vi "大项目框外观 1.vi"(0 "Data In":T4 caption="数据输入", 2 "Display State In":T2 caption="显示状态输入", 3 "Container State":T3 caption="容器状态") -> (6 "Data Out":T4 caption="数据输出", 7 "Display State Out":T2 caption="显示状态输出", 8 "Action":T1 caption="动作")   [LabVIEW 2016, in "大项目框.xctl"]
uses:
  <vilib>/_xctls/Container State.ctl
  <vilib>/_xctls/Action.ctl
  <vilib>/_xctls/XControlSupport.lvlib
panel:
  out "单位":string="mg/L"
  out "浓度":string
  out "英文项目名称":string
  out "中文项目名称":string
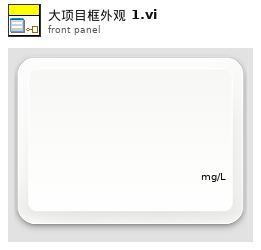
[diagram p1: front panel]
types:
  T1 = typedef "XControlSupport.lvlib/Action.ctl" = cluster{"Data Changed?":bool, "State Changed?":bool, "Action Name":string}
  T2 = typedef "大项目框.xctl/大项目框状态 1.ctl" = cluster{"Numeric":dbl}
  T3 = typedef "XControlSupport.lvlib/Container State.ctl" = cluster{"Indicator?":bool, "Run Mode?":bool, " Refnum":refnum<vi>}
  T4 = typedef "大项目框.xctl/大项目框数据 1.ctl" = cluster{"中文项目名称":string, "英文项目名称":string, "浓度值":string, "单位":string}
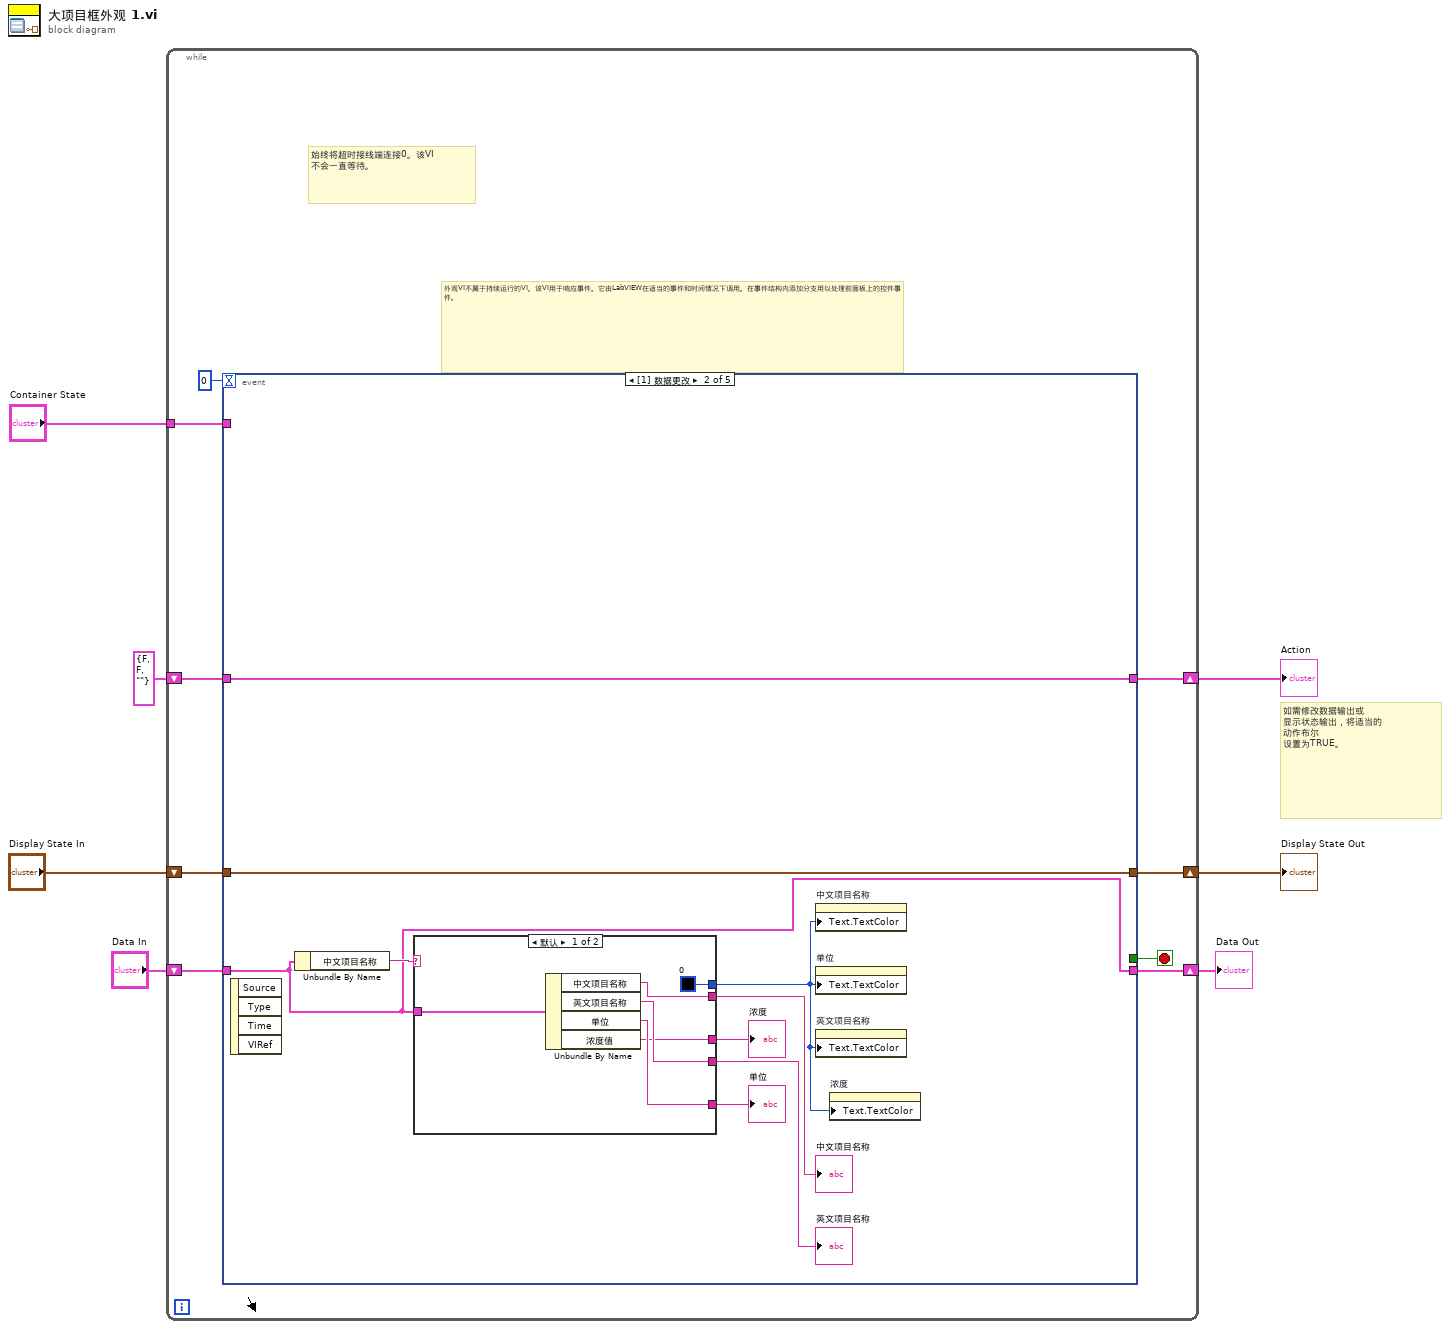
[diagram p0: block diagram]
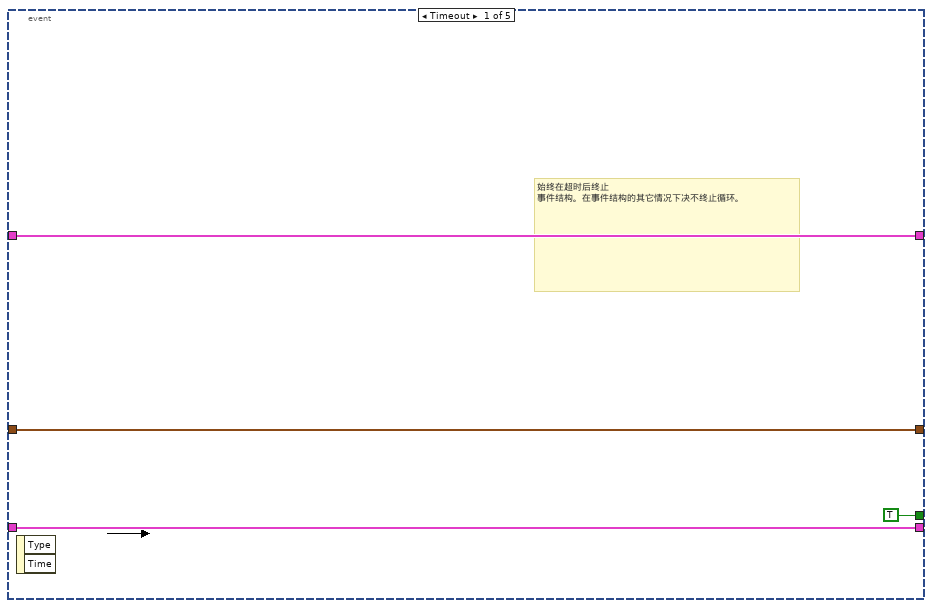
[diagram p2: hidden frame]
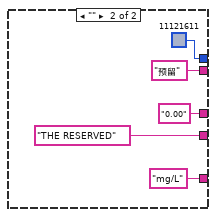
[diagram p3: hidden frame]
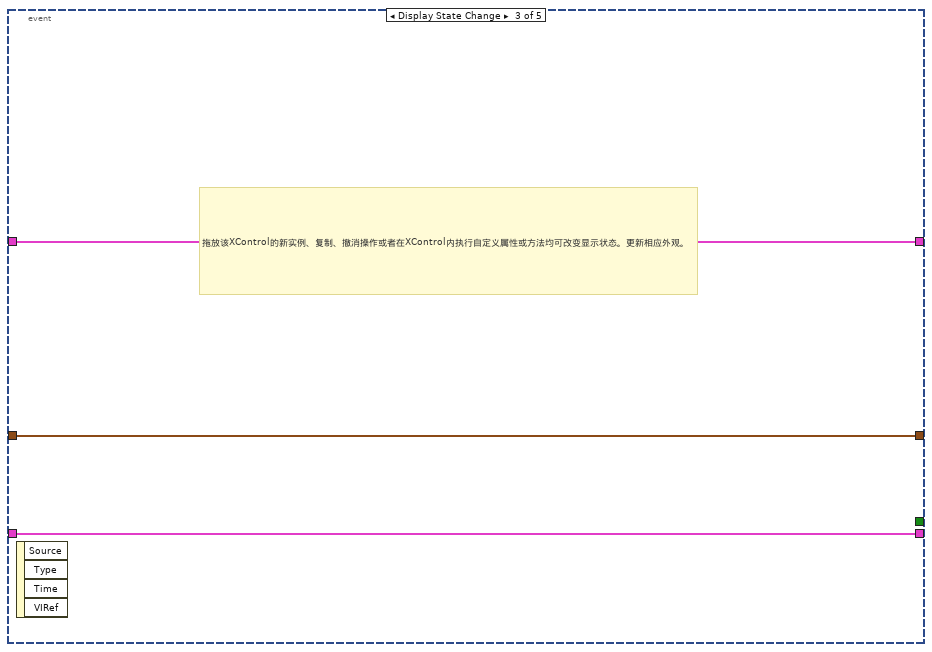
[diagram p4: hidden frame]
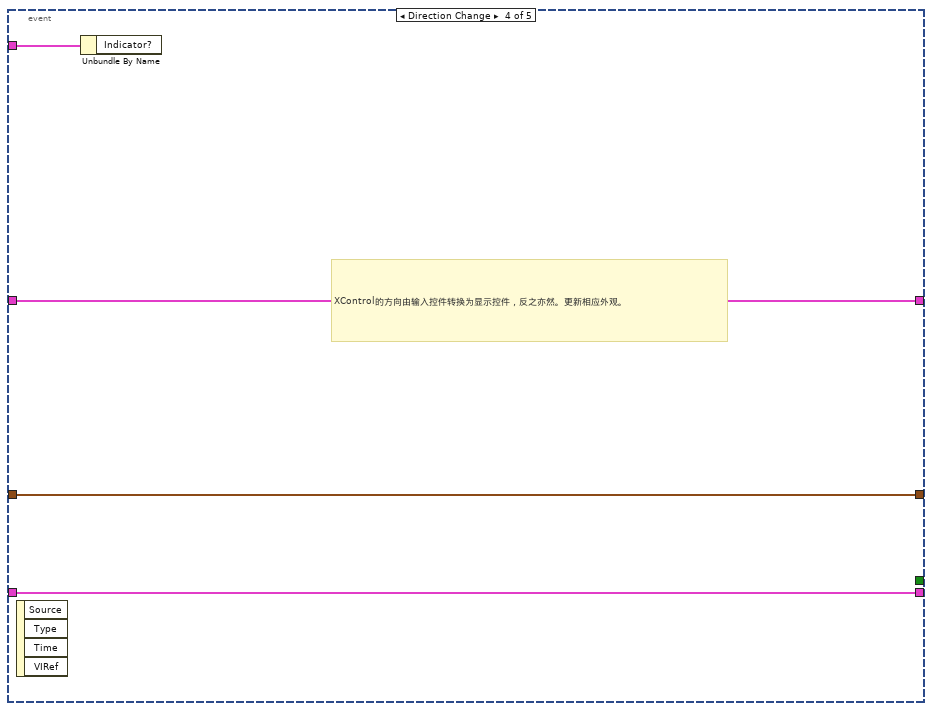
[diagram p5: hidden frame]
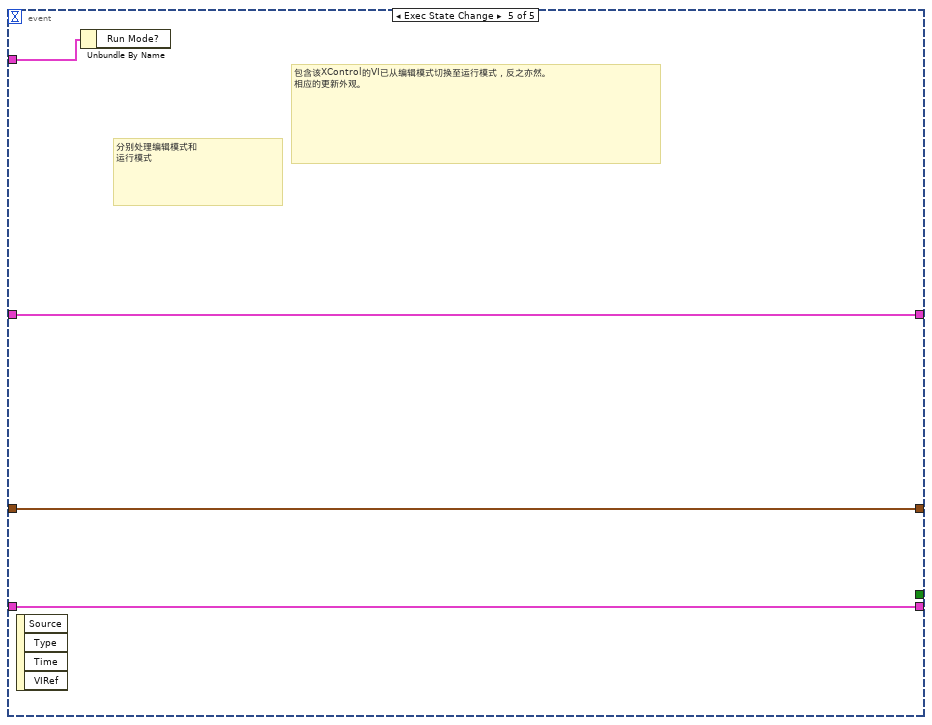
[diagram p6: hidden frame]
diagram:
  # "如需修改数据输出或\n显示状态输出，将适当的\n动作布尔\n设置为TRUE。"
  n1 = while {
    shift-right: [w15] -> w4
    shift-left: "Display State In" -> [w16]
    tunnel: "Container State" -> [w12]
    shift-right: [w10] -> w7
    shift-left: "Data In" -> [w11]
    shift-right: [w8] -> w2
    shift-left: T1 {"Data Changed?"=FALSE, "State Changed?"=FALSE, "Action Name"=""} ("Action") -> [w9]
    stop <- w14 stop-if-true
    # "外观VI不属于持续运行的VI。该VI用于响应事件。它由LabVIEW在适当的事件和时间情况下调用。在事件结构内添加分支用以处理前面板上的控件事件。"
    # "始终将超时接线端连接0。该VI\n不会一直等待。"
    n2 = event shown="[1] 数据更改" {
      selector: _ -> [_ _ _ _ _]
      dyn-events: _ -> [_ _ _ _ _]
      timeout: 0 -> [_ _ _ _ _]
      tunnel: w16 -> [w18 w29 w43 w46 w50]
      tunnel: [w18 w29 w43 w46 w50] -> w15
      tunnel: [TRUE _ _ _ _] -> w14
      tunnel: w12 -> [_ _ _ w47 w51]
      tunnel: w11 -> [w17 w26 w42 w45 w49]
      tunnel: [w17 w26 w42 w45 w49] -> w10
      tunnel: [w19 w28 w41 w44 w48] -> w8
      tunnel: w9 -> [w19 w28 w41 w44 w48]
      event Timeout {
        # "始终在超时后终止\n事件结构。在事件结构的其它情况下决不终止循环。"
        n3 = event-data() -> ()  [unwired: 1 in, 2 out]
      }
      event Data Change {
        n4 = event-data() -> ()  [unwired: 1 in, 4 out]
        n5 = Unbundle By Name(w26) -> ("中文项目名称"=w27:string)
        n6 = case shown="默认" w27 {
          tunnel: w26 -> [w35 _]
          tunnel: [w34 "预留" ("中文项目名称")] -> w23
          tunnel: [w33 "THE RESERVED" ("英文项目名称")] -> w25
          tunnel: [w32 "mg/L" ("单位")] -> w24
          tunnel: [w31 "0.00" ("浓度值")] -> w21
          tunnel: [u32 0 u32 11121611] -> w22
          frame Default {
            n7 = Unbundle By Name(w35) -> ("中文项目名称"=w34:string, "英文项目名称"=w33:string, "单位"=w32:string, "浓度值"=w31:string)
          }
          frame "" {
          }
        }
        "浓度" <- w21
        "中文项目名称" <- w23
        "单位" <- w24
        "英文项目名称" <- w25
        n8 = property on="中文项目名称" class="Str"("Text.TextColor"=w22) -> ()  [unwired: 2 in, 2 out]
        n9 = property on="单位" class="Str"("Text.TextColor"=w22) -> ()  [unwired: 2 in, 2 out]
        n10 = property on="英文项目名称" class="Str"("Text.TextColor"=w22) -> ()  [unwired: 2 in, 2 out]
        n11 = property on="浓度" class="Str"("Text.TextColor"=w22) -> ()  [unwired: 2 in, 2 out]
      }
      event Display State Change {
        # "拖放该XControl的新实例、复制、撤消操作或者在XControl内执行自定义属性或方法均可改变显示状态。更新相应外观。"
        n12 = event-data() -> ()  [unwired: 1 in, 4 out]
      }
      event Direction Change {
        # "XControl的方向由输入控件转换为显示控件，反之亦然。更新相应外观。"
        n13 = event-data() -> ()  [unwired: 1 in, 4 out]
        n14 = Unbundle By Name(w47) -> ()  [unwired: 1 out]
      }
      event Exec State Change {
        # "包含该XControl的VI已从编辑模式切换至运行模式，反之亦然。\n相应的更新外观。"
        # "分别处理编辑模式和\n运行模式"
        n15 = event-data() -> ()  [unwired: 1 in, 4 out]
        n16 = Unbundle By Name(w51) -> ()  [unwired: 1 out]
      }
    }
  }
  "Display State Out" <- w4
  "Data Out" <- w7
  "Action" <- w2
